vi "IPES Pressures.vi"() -> ()   [LabVIEW 2010]
uses:
  <vilib>/Analysis/NI_AALBase.lvlib
panel:
  out "Prep Chamber Ion":dbl format="%#2_4e"
  out "Prep Chamber Conv":dbl format="%#2_4e"
  in  "Tab Control":T1(tab)
  out "Load Lock Backing":dbl format="%#_4e"
  out "Prep Chamber":dbl format="%#2_4e"
  out "Main Chamber":dbl format="%#_4e"
  out "Krypton":dbl format="%#_4e"
  out "Acetone":dbl format="%#_4e"
  in  "End Program":bool caption="(Safe Stop)"
  out "IGC100 Main Status":string
  out "IGC100 Prep Status":string
  in  "Communication Interval (ms)":u32
  in  "Log Interval (s)":u32=1 min=1
  in  "Averaging Time (s)":u32=1
  in  "Enable IGC100 Main":bool=TRUE
  in  "Enable IGC100 Prep":bool=TRUE
  out "IGC100 Prep Online":bool
  out "IGC100 Main Online":bool
  in  "IGC100 Main Port":refnum<visa-resource-name>="COM6"
  in  "IGC100 Prep Port":refnum<visa-resource-name>="COM10"
  out "IGC100 Main error":errorcluster
  out "IGC100 Prep error":errorcluster
  out "QUIT":bool
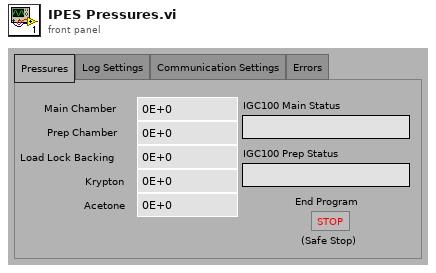
[diagram p1: front panel]
types:
  T1 = enum32{"Pressures", "Log Settings", "Communication Settings", "Errors"}
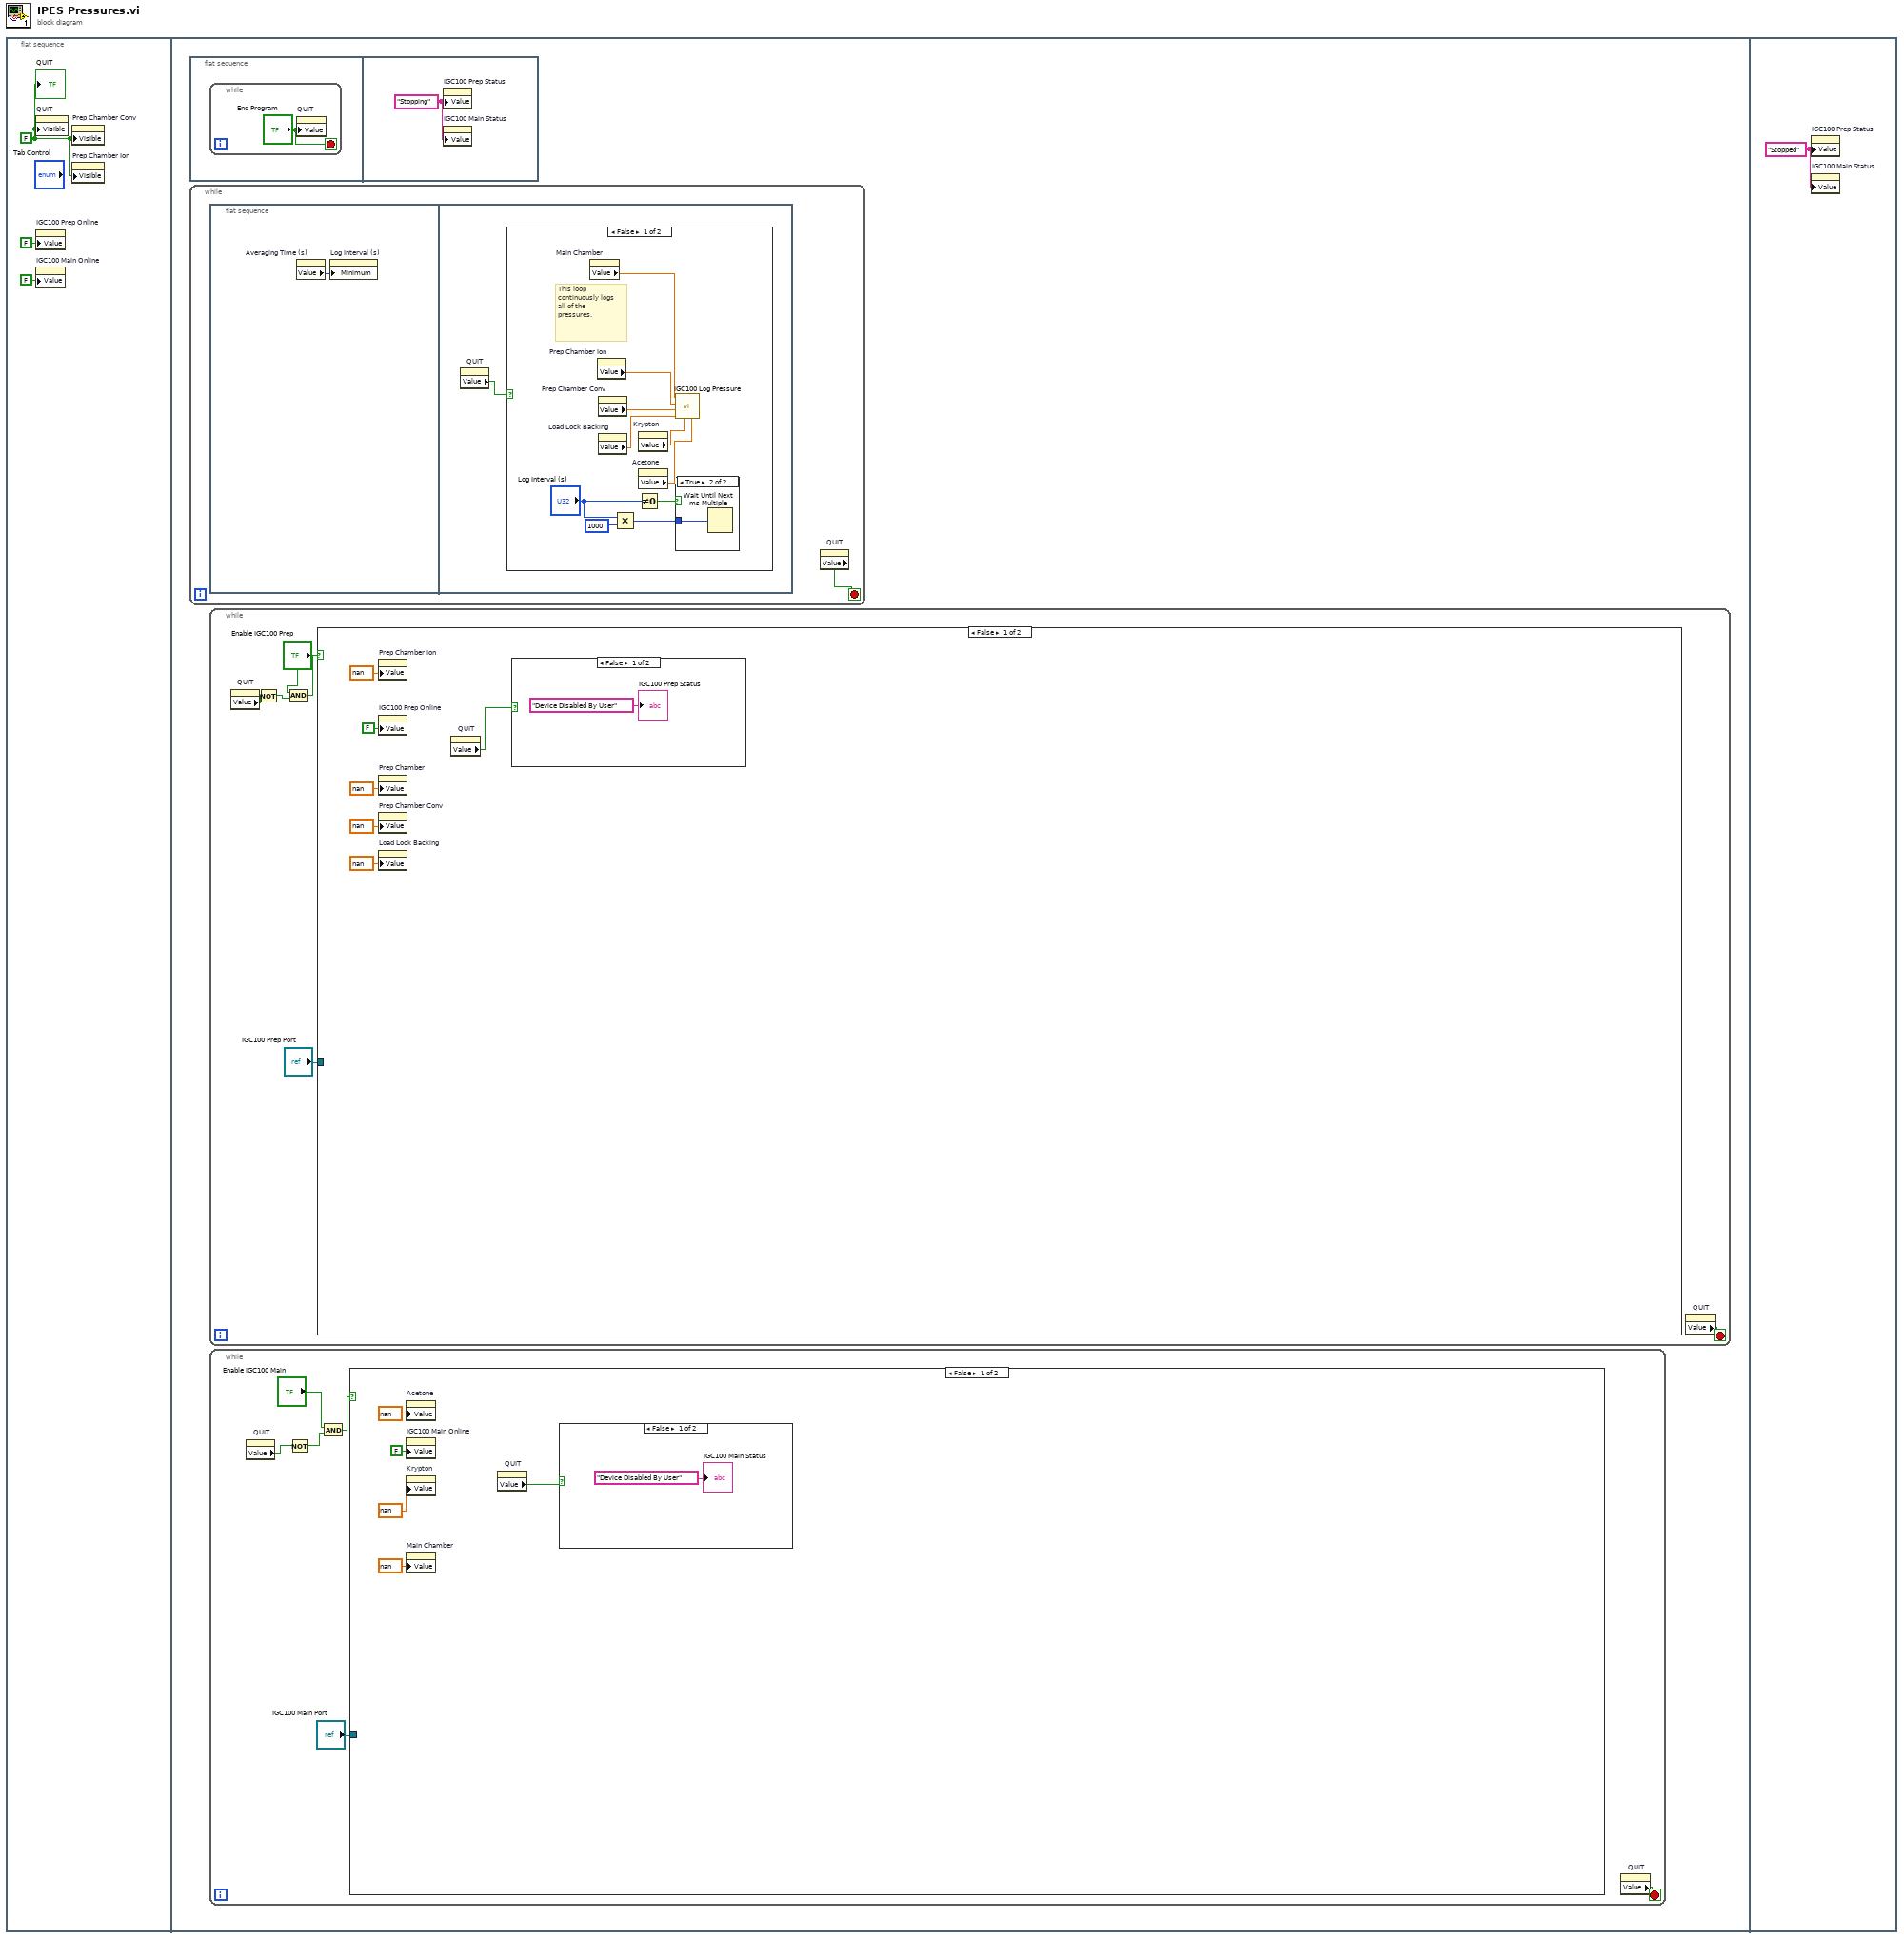
[diagram p0: block diagram]
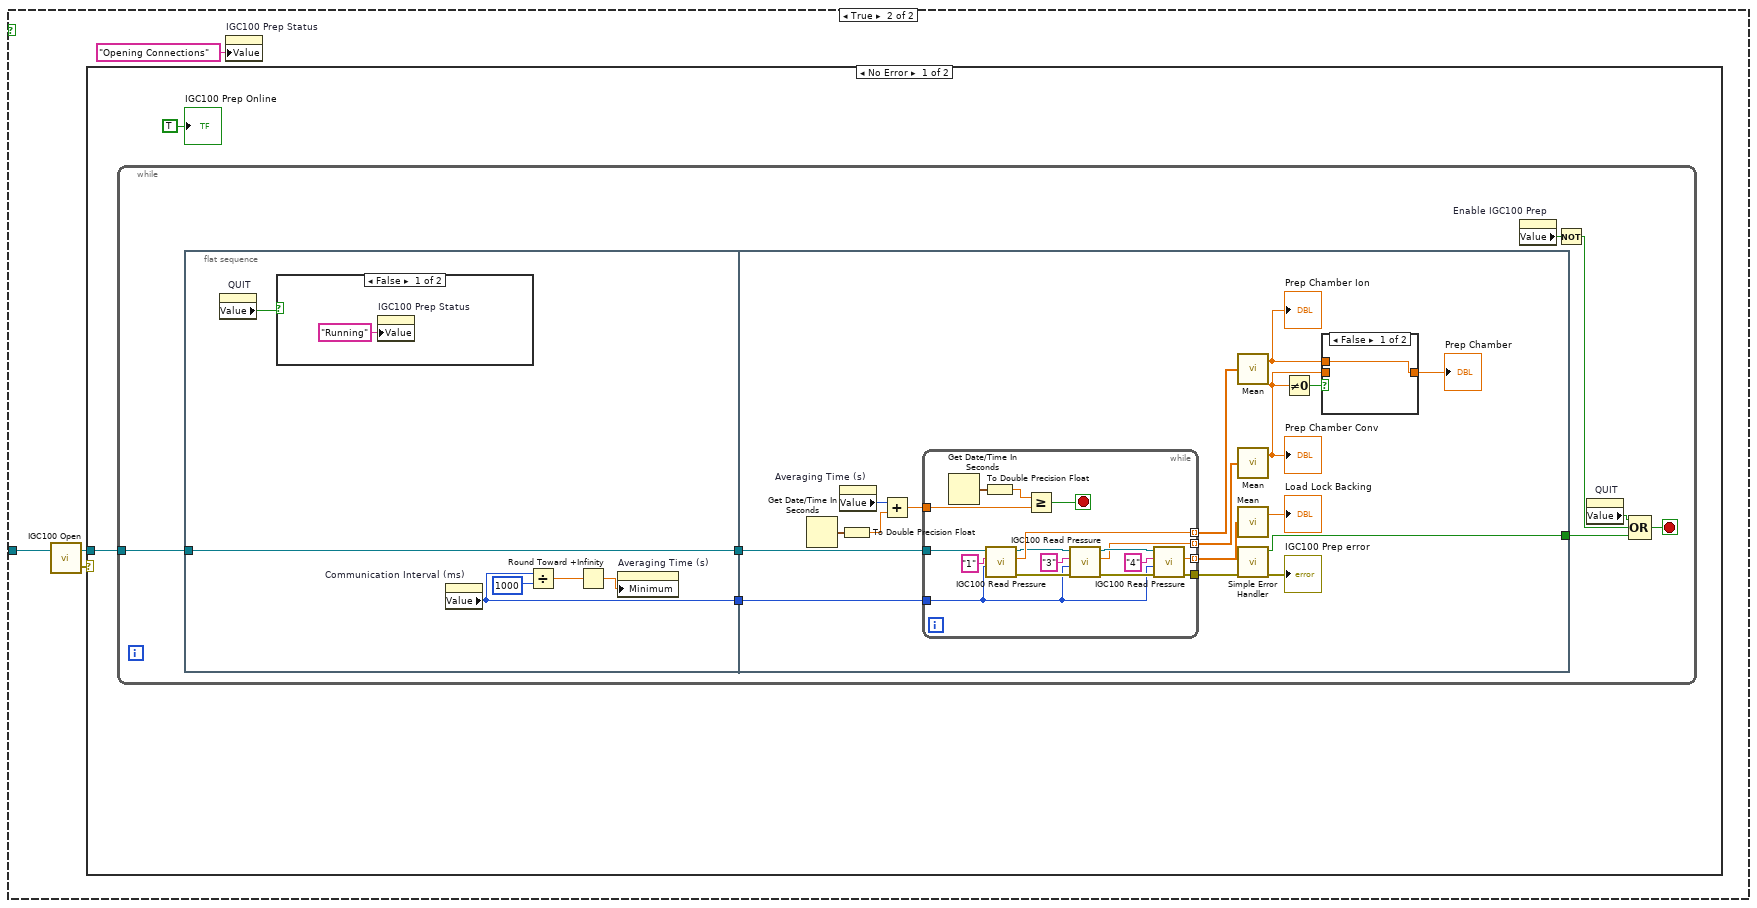
[diagram p5: hidden frame]
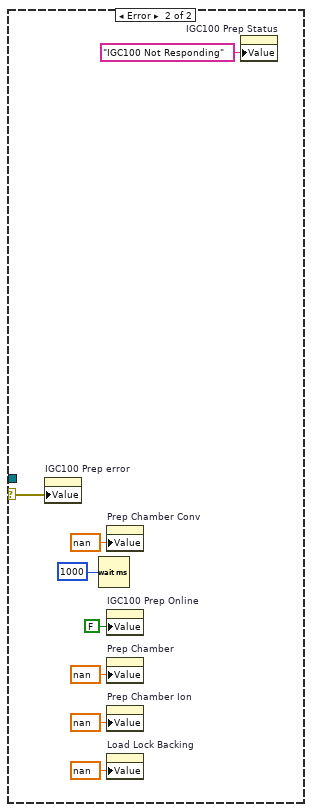
[diagram p8: hidden frame]
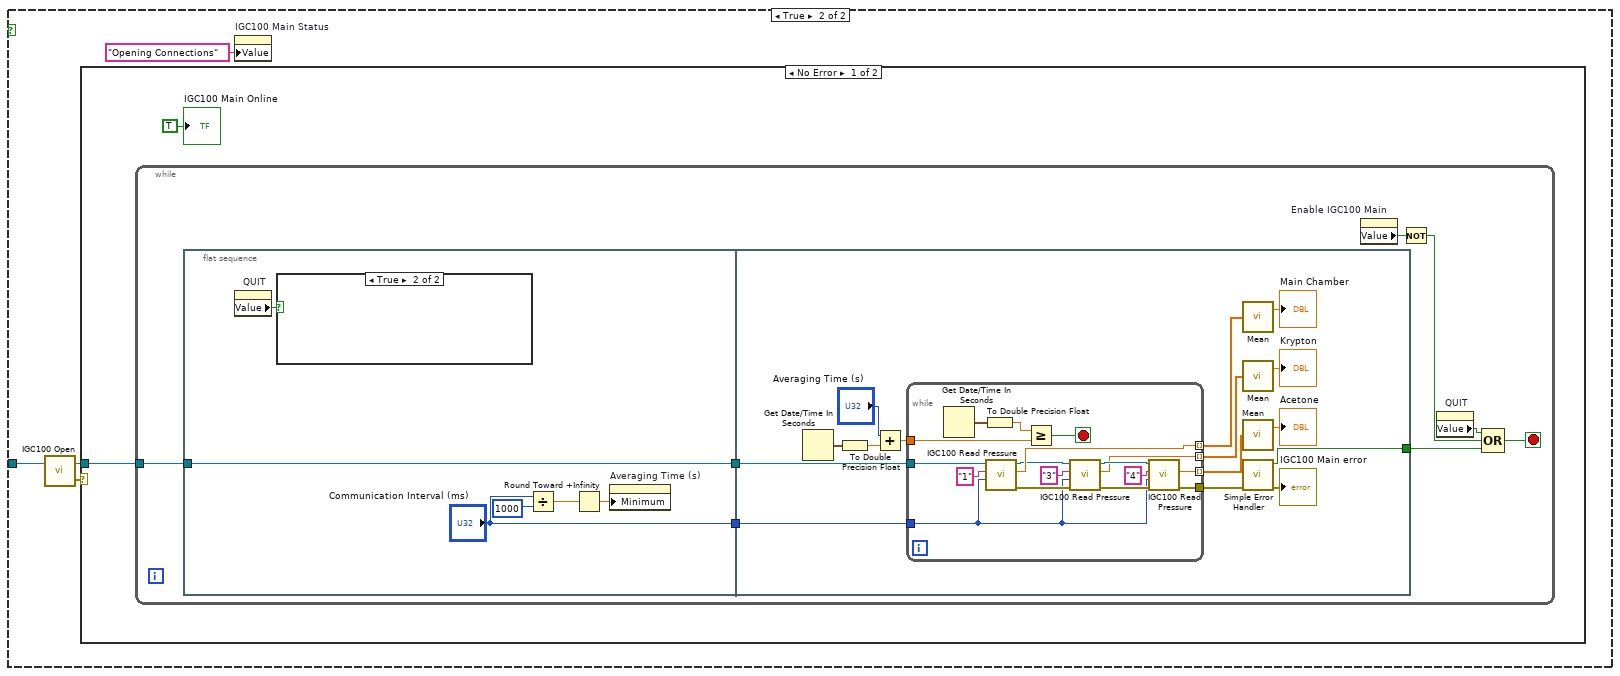
[diagram p10: hidden frame]
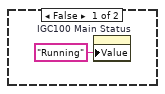
[diagram p11: hidden frame]
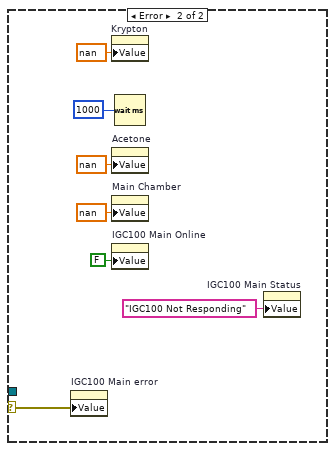
[diagram p12: hidden frame]
diagram:
  n1 = flat-sequence {
    frame #0 {
      w3 = FALSE ("QUIT")
      n2 = property on="QUIT" class="Bool (strict)"("Visible"=w3) -> ()  [unwired: 2 in, 2 out]
      n3 = property on="IGC100 Prep Online" class="Bool (strict)"("Value"=FALSE ("IGC100 Prep Online")) -> ()  [unwired: 2 in, 2 out]
      n4 = property on="IGC100 Main Online" class="Bool (strict)"("Value"=FALSE ("IGC100 Main Online")) -> ()  [unwired: 2 in, 2 out]
      n5 = property on="Prep Chamber Conv" class="DigNum (strict)"("Visible"=w3) -> ()  [unwired: 2 in, 2 out]
      n6 = property on="Prep Chamber Ion" class="DigNum (strict)"("Visible"=w3) -> ()  [unwired: 2 in, 2 out]
      "QUIT" <- w3
    }
    frame #1 {
      n7 = flat-sequence {
        frame #0 {
          n8 = while {
            stop <- "End Program" stop-if-true
            n9 = property on="QUIT" class="Bool (strict)"("Value"="End Program") -> ()  [unwired: 2 in, 2 out]
          }
        }
        frame #1 {
          w5 = "Stopping" ("IGC100 Main Status")
          n10 = property on="IGC100 Prep Status" class="Str"("Value"=w5) -> ()  [unwired: 2 in, 2 out]
          n11 = property on="IGC100 Main Status" class="Str"("Value"=w5) -> ()  [unwired: 2 in, 2 out]
        }
      }
      n12 = while {
        stop <- w6 stop-if-true
        n13 = flat-sequence {
          frame #0 {
            n14 = property on="Averaging Time (s)" class="DigNum (strict)"() -> ("Value"=w7:u32)  [unwired: 2 in, 2 out]
            n15 = property on="Log Interval (s)" class="DigNum (strict)"("Minimum"=w7) -> ()  [unwired: 2 in, 2 out]
          }
          frame #1 {
            n16 = property on="QUIT" class="Bool (strict)"() -> ("Value"=w8:bool)  [unwired: 2 in, 2 out]
            n17 = case shown="False" w8 {
              frame False {
                # "This loop continuously logs all of the pressures."
                n18 = property on="Main Chamber" class="DigNum (strict)"() -> ("Value"=w14:dbl)  [unwired: 2 in, 2 out]
                n19 = property on="Prep Chamber Ion" class="DigNum (strict)"() -> ("Value"=w13:dbl)  [unwired: 2 in, 2 out]
                n20 = property on="Prep Chamber Conv" class="DigNum (strict)"() -> ("Value"=w12:dbl)  [unwired: 2 in, 2 out]
                n21 = property on="Load Lock Backing" class="DigNum (strict)"() -> ("Value"=w11:dbl)  [unwired: 2 in, 2 out]
                n22 = Multiply(x="Log Interval (s)", y=u32 1000) -> (x*y=w15:u32)
                n23 = Not Equal To 0?(x="Log Interval (s)") -> (x != 0?=w18:bool)
                n24 = property on="Krypton" class="DigNum (strict)"() -> ("Value"=w10:dbl)  [unwired: 2 in, 2 out]
                n25 = property on="Acetone" class="DigNum (strict)"() -> ("Value"=w9:dbl)  [unwired: 2 in, 2 out]
                n26 = call "IGC100 Log Pressure.vi"("Acetone (Convectron)"=w9, "Krypton (Convectron)"=w10, "Load Lock Backing Pressure (Convectron)"=w11, "Prep Pressure (Convectron)"=w12, "Prep Pressure (Ion)"=w13, "Main Pressure (Ion)"=w14) -> ()  [unwired: 6 in]
                n27 = case shown="True" w18 {
                  tunnel: w15 -> [_ w19]
                  frame False {
                  }
                  frame True {
                    n28 = Wait Until Next ms Multiple(millisecond multiple=w19) -> ()  [unwired: 1 out]
                  }
                }
              }
              frame True {
              }
            }
          }
        }
        n29 = property on="QUIT" class="Bool (strict)"() -> ("Value"=w6:bool)  [unwired: 2 in, 2 out]
      }
      n30 = while {
        stop <- w24 stop-if-true
        n31 = property on="QUIT" class="Bool (strict)"() -> ("Value"=w20:bool)  [unwired: 2 in, 2 out]
        n32 = Not(x=w20) -> (.not. x?=w21:bool)
        n33 = And(x="Enable IGC100 Prep", y=w21) -> (x .and. y?=w23:bool)
        n34 = case shown="False" w23 {
          tunnel: "IGC100 Prep Port" -> [_ w36]
          frame False {
            n35 = property on="Prep Chamber Ion" class="DigNum (strict)"("Value"=nan ("Prep Chamber Ion")) -> ()  [unwired: 2 in, 2 out]
            n36 = property on="IGC100 Prep Online" class="Bool (strict)"("Value"=FALSE ("IGC100 Prep Online")) -> ()  [unwired: 2 in, 2 out]
            n37 = property on="Prep Chamber" class="DigNum (strict)"("Value"=nan ("Prep Chamber")) -> ()  [unwired: 2 in, 2 out]
            n38 = property on="Prep Chamber Conv" class="DigNum (strict)"("Value"=nan ("Prep Chamber Ion")) -> ()  [unwired: 2 in, 2 out]
            n39 = property on="Load Lock Backing" class="DigNum (strict)"("Value"=nan ("Prep Chamber Ion")) -> ()  [unwired: 2 in, 2 out]
            n40 = property on="QUIT" class="Bool (strict)"() -> ("Value"=w26:bool)  [unwired: 2 in, 2 out]
            n41 = case shown="False" w26 {
              frame False {
                "IGC100 Prep Status" <- "Device Disabled By User" ("IGC100 Main Status")
              }
              frame True {
              }
            }
          }
          frame True {
            n42 = call "IGC100 Open.vi"("VISA in"=w36) -> ("error out"=w34:errorcluster, "VISA out"=w35:refnum<visa-resource-name>)  [unwired: 1 in]
            n43 = case shown="No Error" w34 {
              selector: w34 -> [_ w92]
              tunnel: w35 -> [w38 _]
              frame No Error {
                n44 = while {
                  tunnel: w38 -> [w46]
                  stop <- w42 stop-if-true
                  n45 = flat-sequence {
                    tunnel: w46 -> [w52]
                    tunnel: [w52] -> w40
                    tunnel: [w49] -> w39
                    tunnel: [w62] -> w41
                    tunnel: w40 -> [w70]
                    tunnel: w39 -> [w54]
                    frame #0 {
                      n46 = property on="QUIT" class="Bool (strict)"() -> ("Value"=w47:bool)  [unwired: 2 in, 2 out]
                      n47 = case shown="False" w47 {
                        frame False {
                          n48 = property on="IGC100 Prep Status" class="Str"("Value"="Running" ("IGC100 Main Status")) -> ()  [unwired: 2 in, 2 out]
                        }
                        frame True {
                        }
                      }
                      n49 = property on="Communication Interval (ms)" class="DigNum (strict)"() -> ("Value"=w49:u32)  [unwired: 2 in, 2 out]
                      n50 = Divide(x=w49, y=u32 1000) -> (x/y=w50:dbl)
                      n51 = Round Toward +Infinity(x=w50) -> (ceil(x): smallest int >= x=w51:dbl)
                      n52 = property on="Averaging Time (s)" class="DigNum (strict)"("Minimum"=w51) -> ()  [unwired: 2 in, 2 out]
                    }
                    frame #1 {
                      n53 = Get Date/Time In Seconds() -> (seconds since 1Jan1904=w69:timestamp)
                      n54 = property on="Averaging Time (s)" class="DigNum (strict)"() -> ("Value"=w61:u32)  [unwired: 2 in, 2 out]
                      n55 = To Double Precision Float(number=w69) -> (double precision float=w68:dbl)
                      n56 = Add(x=w61, y=w68) -> (x+y=w67:dbl)
                      n57 = while {
                        tunnel: w70 -> [w89]
                        tunnel: [w87] -> w66 mode=indexing
                        tunnel: w67 -> [w84]
                        tunnel: [w76] -> w65 mode=indexing
                        tunnel: [w75] -> w64 mode=indexing
                        tunnel: [w74] -> w63
                        tunnel: w54 -> [w73]
                        stop <- w83 stop-if-true
                        n58 = Get Date/Time In Seconds() -> (seconds since 1Jan1904=w86:timestamp)
                        n59 = To Double Precision Float(number=w86) -> (double precision float=w85:dbl)
                        n60 = call "IGC100 Read Pressure.vi"("Communication Interval (ms)"=w73, "Channel"="1", "VISA in"=w89) -> ("error out"=w78:errorcluster, "Pressure"=w87:dbl, "VISA out"=w82:refnum<visa-resource-name>)  [unwired: 2 in]
                        n61 = Greater Or Equal?(x=w85, y=w84) -> (x >= y?=w83:bool)
                        n62 = call "IGC100 Read Pressure.vi"("error in"=w78, "Communication Interval (ms)"=w73, "Channel"="3", "VISA in"=w82) -> ("error out"=w77:errorcluster, "Pressure"=w76:dbl, "VISA out"=w81:refnum<visa-resource-name>)  [unwired: 1 in]
                        n63 = call "IGC100 Read Pressure.vi"("error in"=w77, "Communication Interval (ms)"=w73, "Channel"="4", "VISA in"=w81) -> ("error out"=w74:errorcluster, "Pressure"=w75:dbl)  [unwired: 1 in, 1 out]
                      }
                      n64 = call <vilib>:"Mean.vi"("X"=w66) -> ("mean"=w56:dbl)  [unwired: 1 out]
                      "Prep Chamber Ion" <- w56
                      n65 = call <vilib>:"Mean.vi"("X"=w65) -> ("mean"=w57:dbl)  [unwired: 1 out]
                      "Prep Chamber Conv" <- w57
                      n66 = call <vilib>:"Mean.vi"("X"=w64) -> ("mean"=→"Load Lock Backing":dbl)  [unwired: 1 out]
                      n67 = call <vilib>:"Simple Error Handler.vi"("error in (no error)"=w63) -> ("error?"=w62:bool, "error out"=→"IGC100 Prep error":errorcluster)  [unwired: 4 in, 3 out]
                      n68 = Not Equal To 0?(x=w57) -> (x != 0?=w59:bool)
                      n69 = case shown="False" w59 {
                        tunnel: [w71 w72] -> w58
                        tunnel: w57 -> [_ w72]
                        tunnel: w56 -> [w71 _]
                        frame False {
                        }
                        frame True {
                        }
                      }
                      "Prep Chamber" <- w58
                    }
                  }
                  n70 = property on="Enable IGC100 Prep" class="Bool (strict)"() -> ("Value"=w44:bool)  [unwired: 2 in, 2 out]
                  n71 = Not(x=w44) -> (.not. x?=w43:bool)
                  n72 = property on="QUIT" class="Bool (strict)"() -> ("Value"=w45:bool)  [unwired: 2 in, 2 out]
                  n73 = Compound Arithmetic op=OR(w45, w43, w41) -> (w42:bool)
                }
                "IGC100 Prep Online" <- TRUE ("IGC100 Prep Online")
              }
              frame Error {
                n74 = property on="IGC100 Prep error" class="Clust (strict)"("Value"=w92) -> ()  [unwired: 2 in, 2 out]
                n75 = Wait (ms)(milliseconds to wait=u32 1000) -> ()  [unwired: 1 out]
                n76 = property on="Prep Chamber Conv" class="DigNum (strict)"("Value"=nan ("Prep Chamber Ion")) -> ()  [unwired: 2 in, 2 out]
                n77 = property on="IGC100 Prep Online" class="Bool (strict)"("Value"=FALSE ("IGC100 Prep Online")) -> ()  [unwired: 2 in, 2 out]
                n78 = property on="Prep Chamber" class="DigNum (strict)"("Value"=nan ("Prep Chamber")) -> ()  [unwired: 2 in, 2 out]
                n79 = property on="Prep Chamber Ion" class="DigNum (strict)"("Value"=nan ("Prep Chamber Ion")) -> ()  [unwired: 2 in, 2 out]
                n80 = property on="Load Lock Backing" class="DigNum (strict)"("Value"=nan ("Prep Chamber Ion")) -> ()  [unwired: 2 in, 2 out]
                n81 = property on="IGC100 Prep Status" class="Str"("Value"="IGC100 Not Responding" ("IGC100 Main Status")) -> ()  [unwired: 2 in, 2 out]
              }
            }
            n82 = property on="IGC100 Prep Status" class="Str"("Value"="Opening Connections" ("IGC100 Main Status")) -> ()  [unwired: 2 in, 2 out]
          }
        }
        n83 = property on="QUIT" class="Bool (strict)"() -> ("Value"=w24:bool)  [unwired: 2 in, 2 out]
      }
      n84 = while {
        stop <- w103 stop-if-true
        n85 = property on="QUIT" class="Bool (strict)"() -> ("Value"=w98:bool)  [unwired: 2 in, 2 out]
        n86 = Not(x=w98) -> (.not. x?=w99:bool)
        n87 = And(x="Enable IGC100 Main", y=w99) -> (x .and. y?=w101:bool)
        n88 = case shown="False" w101 {
          tunnel: "IGC100 Main Port" -> [_ w112]
          frame False {
            n89 = property on="Acetone" class="DigNum (strict)"("Value"=nan ("Acetone")) -> ()  [unwired: 2 in, 2 out]
            n90 = property on="IGC100 Main Online" class="Bool (strict)"("Value"=FALSE ("IGC100 Main Online")) -> ()  [unwired: 2 in, 2 out]
            n91 = property on="Krypton" class="DigNum (strict)"("Value"=nan ("Krypton")) -> ()  [unwired: 2 in, 2 out]
            n92 = property on="Main Chamber" class="DigNum (strict)"("Value"=nan ("Main Chamber")) -> ()  [unwired: 2 in, 2 out]
            n93 = property on="QUIT" class="Bool (strict)"() -> ("Value"=w104:bool)  [unwired: 2 in, 2 out]
            n94 = case shown="False" w104 {
              frame False {
                "IGC100 Main Status" <- "Device Disabled By User" ("IGC100 Main Status")
              }
              frame True {
              }
            }
          }
          frame True {
            n95 = call "IGC100 Open.vi"("VISA in"=w112) -> ("error out"=w110:errorcluster, "VISA out"=w111:refnum<visa-resource-name>)  [unwired: 1 in]
            n96 = case shown="No Error" w110 {
              selector: w110 -> [_ w164]
              tunnel: w111 -> [w115 _]
              frame No Error {
                n97 = while {
                  tunnel: w115 -> [w123]
                  stop <- w122 stop-if-true
                  n98 = flat-sequence {
                    tunnel: w123 -> [w129]
                    tunnel: [w129] -> w120
                    tunnel: ["Communication Interval (ms)"] -> w119
                    tunnel: [w134] -> w121
                    tunnel: w120 -> [w145]
                    tunnel: w119 -> [w131]
                    frame #0 {
                      n99 = property on="QUIT" class="Bool (strict)"() -> ("Value"=w124:bool)  [unwired: 2 in, 2 out]
                      n100 = case shown="True" w124 {
                        frame False {
                          n101 = property on="IGC100 Main Status" class="Str"("Value"="Running" ("IGC100 Main Status")) -> ()  [unwired: 2 in, 2 out]
                        }
                        frame True {
                        }
                      }
                      n102 = Divide(x="Communication Interval (ms)", y=u32 1000) -> (x/y=w127:dbl)
                      n103 = Round Toward +Infinity(x=w127) -> (ceil(x): smallest int >= x=w128:dbl)
                      n104 = property on="Averaging Time (s)" class="DigNum (strict)"("Minimum"=w128) -> ()  [unwired: 2 in, 2 out]
                    }
                    frame #1 {
                      n105 = Get Date/Time In Seconds() -> (seconds since 1Jan1904=w144:timestamp)
                      n106 = To Double Precision Float(number=w144) -> (double precision float=w143:dbl)
                      n107 = Add(x="Averaging Time (s)", y=w143) -> (x+y=w142:dbl)
                      n108 = while {
                        tunnel: w145 -> [w162]
                        tunnel: [w160] -> w141 mode=indexing
                        tunnel: w142 -> [w157]
                        tunnel: [w149] -> w140 mode=indexing
                        tunnel: [w148] -> w139 mode=indexing
                        tunnel: [w147] -> w135
                        tunnel: w131 -> [w146]
                        stop <- w156 stop-if-true
                        n109 = Get Date/Time In Seconds() -> (seconds since 1Jan1904=w159:timestamp)
                        n110 = To Double Precision Float(number=w159) -> (double precision float=w158:dbl)
                        n111 = call "IGC100 Read Pressure.vi"("Communication Interval (ms)"=w146, "Channel"="1", "VISA in"=w162) -> ("error out"=w151:errorcluster, "Pressure"=w160:dbl, "VISA out"=w155:refnum<visa-resource-name>)  [unwired: 2 in]
                        n112 = Greater Or Equal?(x=w158, y=w157) -> (x >= y?=w156:bool)
                        n113 = call "IGC100 Read Pressure.vi"("error in"=w151, "Communication Interval (ms)"=w146, "Channel"="3", "VISA in"=w155) -> ("error out"=w150:errorcluster, "Pressure"=w149:dbl, "VISA out"=w154:refnum<visa-resource-name>)  [unwired: 1 in]
                        n114 = call "IGC100 Read Pressure.vi"("error in"=w150, "Communication Interval (ms)"=w146, "Channel"="4", "VISA in"=w154) -> ("error out"=w147:errorcluster, "Pressure"=w148:dbl)  [unwired: 1 in, 1 out]
                      }
                      n115 = call <vilib>:"Mean.vi"("X"=w141) -> ("mean"=→"Main Chamber":dbl)  [unwired: 1 out]
                      n116 = call <vilib>:"Mean.vi"("X"=w140) -> ("mean"=→"Krypton":dbl)  [unwired: 1 out]
                      n117 = call <vilib>:"Mean.vi"("X"=w139) -> ("mean"=→"Acetone":dbl)  [unwired: 1 out]
                      n118 = call <vilib>:"Simple Error Handler.vi"("error in (no error)"=w135) -> ("error?"=w134:bool, "error out"=→"IGC100 Main error":errorcluster)  [unwired: 4 in, 3 out]
                    }
                  }
                  n119 = property on="Enable IGC100 Main" class="Bool (strict)"() -> ("Value"=w116:bool)  [unwired: 2 in, 2 out]
                  n120 = Not(x=w116) -> (.not. x?=w117:bool)
                  n121 = property on="QUIT" class="Bool (strict)"() -> ("Value"=w118:bool)  [unwired: 2 in, 2 out]
                  n122 = Compound Arithmetic op=OR(w118, w117, w121) -> (w122:bool)
                }
                "IGC100 Main Online" <- TRUE ("IGC100 Main Online")
              }
              frame Error {
                n123 = property on="IGC100 Main error" class="Clust (strict)"("Value"=w164) -> ()  [unwired: 2 in, 2 out]
                n124 = property on="Krypton" class="DigNum (strict)"("Value"=nan ("Krypton")) -> ()  [unwired: 2 in, 2 out]
                n125 = property on="Acetone" class="DigNum (strict)"("Value"=nan ("Acetone")) -> ()  [unwired: 2 in, 2 out]
                n126 = property on="Main Chamber" class="DigNum (strict)"("Value"=nan ("Main Chamber")) -> ()  [unwired: 2 in, 2 out]
                n127 = property on="IGC100 Main Online" class="Bool (strict)"("Value"=FALSE ("IGC100 Main Online")) -> ()  [unwired: 2 in, 2 out]
                n128 = Wait (ms)(milliseconds to wait=u32 1000) -> ()  [unwired: 1 out]
                n129 = property on="IGC100 Main Status" class="Str"("Value"="IGC100 Not Responding" ("IGC100 Main Status")) -> ()  [unwired: 2 in, 2 out]
              }
            }
            n130 = property on="IGC100 Main Status" class="Str"("Value"="Opening Connections" ("IGC100 Main Status")) -> ()  [unwired: 2 in, 2 out]
          }
        }
        n131 = property on="QUIT" class="Bool (strict)"() -> ("Value"=w103:bool)  [unwired: 2 in, 2 out]
      }
    }
    frame #2 {
      w170 = "Stopped" ("IGC100 Main Status")
      n132 = property on="IGC100 Prep Status" class="Str"("Value"=w170) -> ()  [unwired: 2 in, 2 out]
      n133 = property on="IGC100 Main Status" class="Str"("Value"=w170) -> ()  [unwired: 2 in, 2 out]
    }
  }
